vi "RawXMLToPrefSet.vi"(8 "error in (no error)":errorcluster, 10 "path to XML document":path, 11 "Preferences in":refnum<class "SetListPrefs.lvclass">) -> (0 "error out":errorcluster, 3 "Preferences out":refnum<class "SetListPrefs.lvclass">)   [LabVIEW 2013, in "SetListPrefs.lvclass"]
uses:
  SetListPrefs.lvclass
  <vilib>/xml/NI_XML.lvlib
  <vilib>/xml/Close Reference(Node).vi
  <resource>/objmgr/DOMUserDefRef.rc
  <vilib>/Utility/error.llb/DialogType.ctl
  <vilib>/xml/Load XML File.vi
panel:
  out "XML":string
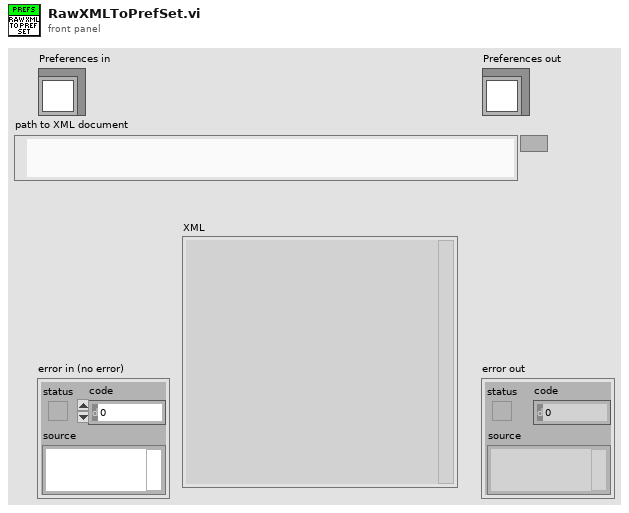
[diagram p1: front panel]
types:
  T1 = typedef "DialogType.ctl" = u16
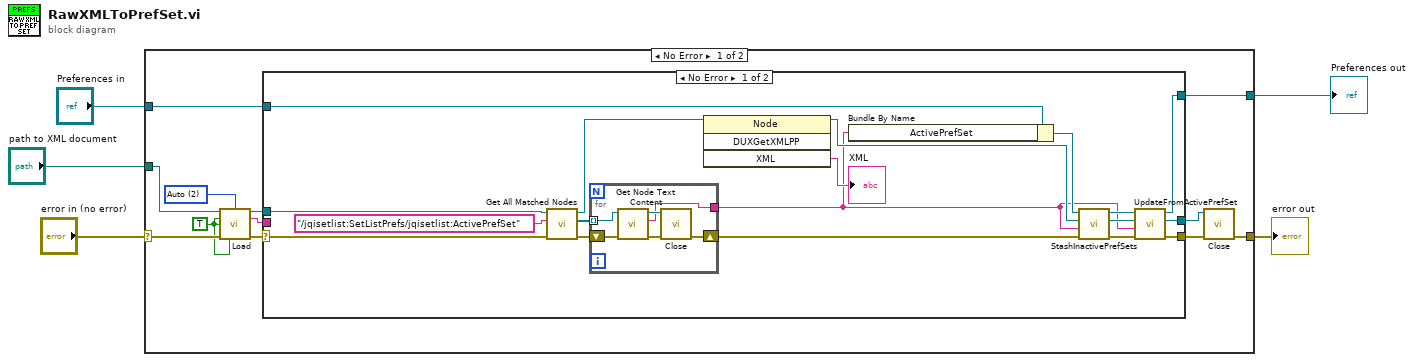
[diagram p0: block diagram]
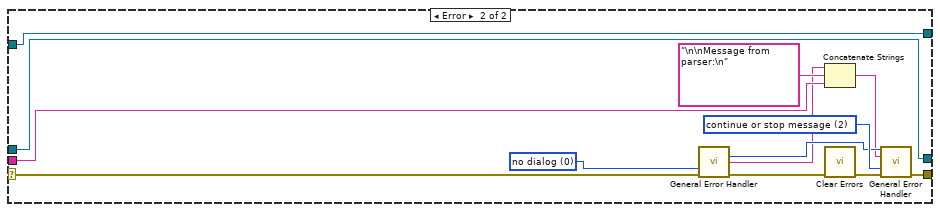
[diagram p2: hidden frame]
diagram:
  n1 = case shown="No Error" "error in (no error)" {
    selector: "error in (no error)" -> [w11 w56]
    tunnel: [w9 w56] -> w4
    tunnel: [w10 w55] -> w2
    tunnel: "Preferences in" -> [w12 w55]
    tunnel: "path to XML document" -> [w7 _]
    frame No Error {
      w6 = 2 items=["Never", "Always", "Auto"] ("validate on load (Auto)")
      w8 = TRUE ("process namespaces (False)")
      n2 = call-poly <vilib>:"Load.vi"("path to XML document"=w7, "validate on load (Auto)"=w6, "process namespaces (False)"=w8, "process schema (False)"=w8, "error in (no error)"=w11, "schema full checking (False)"=w8) -> ("DOM document out"=w13:refnum<k20>, "parse errors"=w17:string, "error out"=w16:errorcluster)  [unwired: 7 in]
      n3 = case shown="No Error" w16 {
        selector: w16 -> [w34 w54]
        tunnel: w13 -> [w33 w46]
        tunnel: [w26 w46] -> w14
        tunnel: [w27 w48] -> w15
        tunnel: w12 -> [w28 w47]
        tunnel: [w18 w47] -> w10
        tunnel: w17 -> [_ w51]
        frame No Error {
          n4 = call <vilib>:"Get All Matched Nodes.vi"("error in (no error)"=w34, "XPath expression"="/jqisetlist:SetListPrefs/jqisetlist:ActivePrefSet", "node in"=w33) -> ("error out"=w31:errorcluster, "node result array"=w30:refnum<k20>[], "node out"=w29:refnum<k20>)  [unwired: 6 in]
          n5 = for {
            shift-right: [w36] -> w20
            shift-left: w31 -> [w41]
            tunnel: w30 -> [w38] mode=indexing
            tunnel: [w37] -> w19
            n6 = call <vilib>:"Get Node Text Content.vi"("error in (no error)"=w41, "node in"=w38) -> ("error out"=w40:errorcluster, "node text"=w37:string, "node out"=w39:refnum<k20>)  [unwired: 7 in]
            n7 = call-poly <vilib>:"Close.vi"("error in (no error)"=w40, "node"=w39) -> ("error out"=w36:errorcluster)  [unwired: 7 in]
          }
          n8 = invoke class="Node" method="DUXGetXMLPP"(reference=w29) -> (reference out=w22:refnum<k20>, "XML"=→"XML":string)  [unwired: 3 in, 2 out]
          n9 = Bundle By Name(cluster=w28, "ActivePrefSet"=w19) -> (w25:refnum<class "SetListPrefs.lvclass">)
          n10 = call "StashInactivePrefSets.vi"("error in (no error)"=w20, "Active PrefSet"=w19, "node in"=w22, "Preferences in"=w25) -> ("error out"=w21:errorcluster, "node out"=w23:refnum<k20>, "Preferences out"=w24:refnum<class "SetListPrefs.lvclass">)  [unwired: 5 in]
          n11 = call "UpdateFromActivePrefSet.vi"("error in (no error)"=w21, "Active PrefSet"=w19, "node in"=w23, "Preferences in"=w24) -> ("error out"=w27:errorcluster, "node out"=w26:refnum<k20>, "Preferences out"=w18:refnum<class "SetListPrefs.lvclass">)  [unwired: 5 in]
        }
        frame Error {
          w45 = T1 2 items=["no dialog", "OK message", "continue or stop message", "OK message + warnings", "continue/stop + warnings"] ("type of dialog (OK msg:1)")
          w53 = T1 0 items=["no dialog", "OK message", "continue or stop message", "OK message + warnings", "continue/stop + warnings"] ("type of dialog (OK msg:1)")
          n12 = call <vilib>:"General Error Handler.vi"("type of dialog (OK msg:1)"=w53, "error in (no error)"=w54) -> ("code out"=w44:i32, "source out"=w43:string, "error out"=w50:errorcluster)  [unwired: 9 in, 2 out]
          n13 = Concatenate Strings(w43, "\n\nMessage from parser:\n" ("string"), w51) -> (w42:string)
          n14 = call <vilib>:"Clear Errors.vi"("error in (no error)"=w50) -> ("error out"=w49:errorcluster)  [unwired: 6 in]
          n15 = call <vilib>:"General Error Handler.vi"("[error code] (0)"=w44, "[error source] (\" \")"=w42, "type of dialog (OK msg:1)"=w45, "error in (no error)"=w49) -> ("error out"=w48:errorcluster)  [unwired: 7 in, 4 out]
        }
      }
      n16 = call-poly <vilib>:"Close.vi"("error in (no error)"=w15, "node"=w14) -> ("error out"=w9:errorcluster)  [unwired: 7 in]
    }
    frame Error {
    }
  }
  "error out" <- w4
  "Preferences out" <- w2
